vi "Main.vi"() -> ()   [LabVIEW 2024]
doc: "Aplikacja służąca do autoryzacji dostępu oparta na biometrycznej weryfikacji tożsamości"
uses:
  <vilib>/userDefined/High Color/IMAQdx.ctl
  <vilib>/vision/Image Controls.llb/IMAQ Image.ctl
  <vilib>/vision/driver/NI_Vision_Acquisition_Software.lvlib
panel:
  in  "Exit Application":bool caption="Click to terminate the application"
  in  "Tab Control":enum32{"Page 1", "Page 2", "Page 3", "Page 4"}(tab)
  in  "OK Button":bool
  out "Image Display":T1(plugin-control)
  in  "Input":string
  in  "Manage input data":bool
  in  "Add user":bool
  out "UserName":string
  out "Image Display 2":T1(plugin-control)
  in  "Save biometrics":bool
  in  "Name":string
  in  "Surname":string
  # "Processing..."
  # "Welcome"
  # "to control Panel"
  # "Now you can choose what you want to do"
  # "Simple input manager"
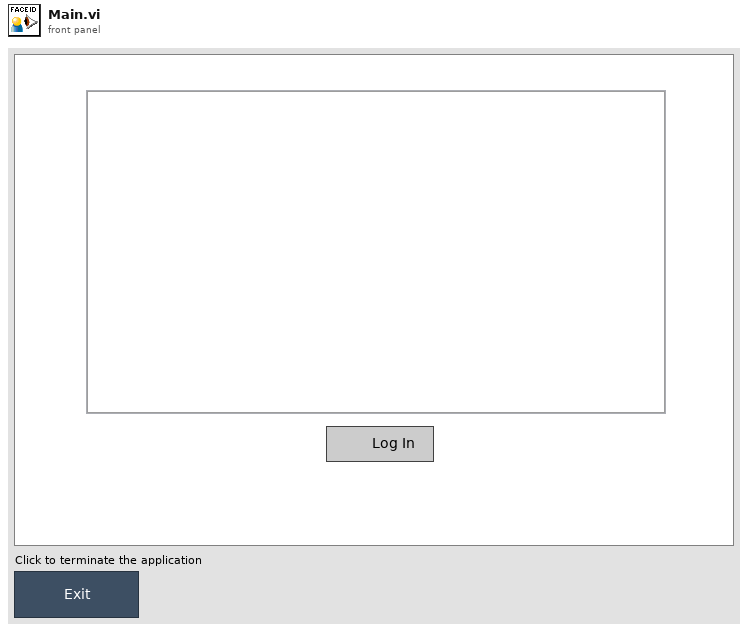
[diagram p1: front panel]
types:
  T1 = typedef "IMAQ Image.ctl" = refnum<image>
  T2 = enum32{"Invalid", "Standard", "Closed", "Hidden", "Minimized", "Maximized"}
  T3 = enum32{"invalid app kind", "Development System", "Run Time System", "Student Edition", "Embedded LabVIEW", "Evaluation", "Custom"}
  T4 = typedef "IMAQdx.ctl" = refnum<k21>
  T5 = cluster{"Core":cluster{"Current VI Reference":refnum<vi>, "Close Panel on Exit?":bool}, "New Image":T1, "IMAQdx Session":T4, "Img Path":string, "NameDisplay":string}
  T6 = cluster{"Current VI Reference":refnum<vi>, "Close Panel on Exit?":bool}
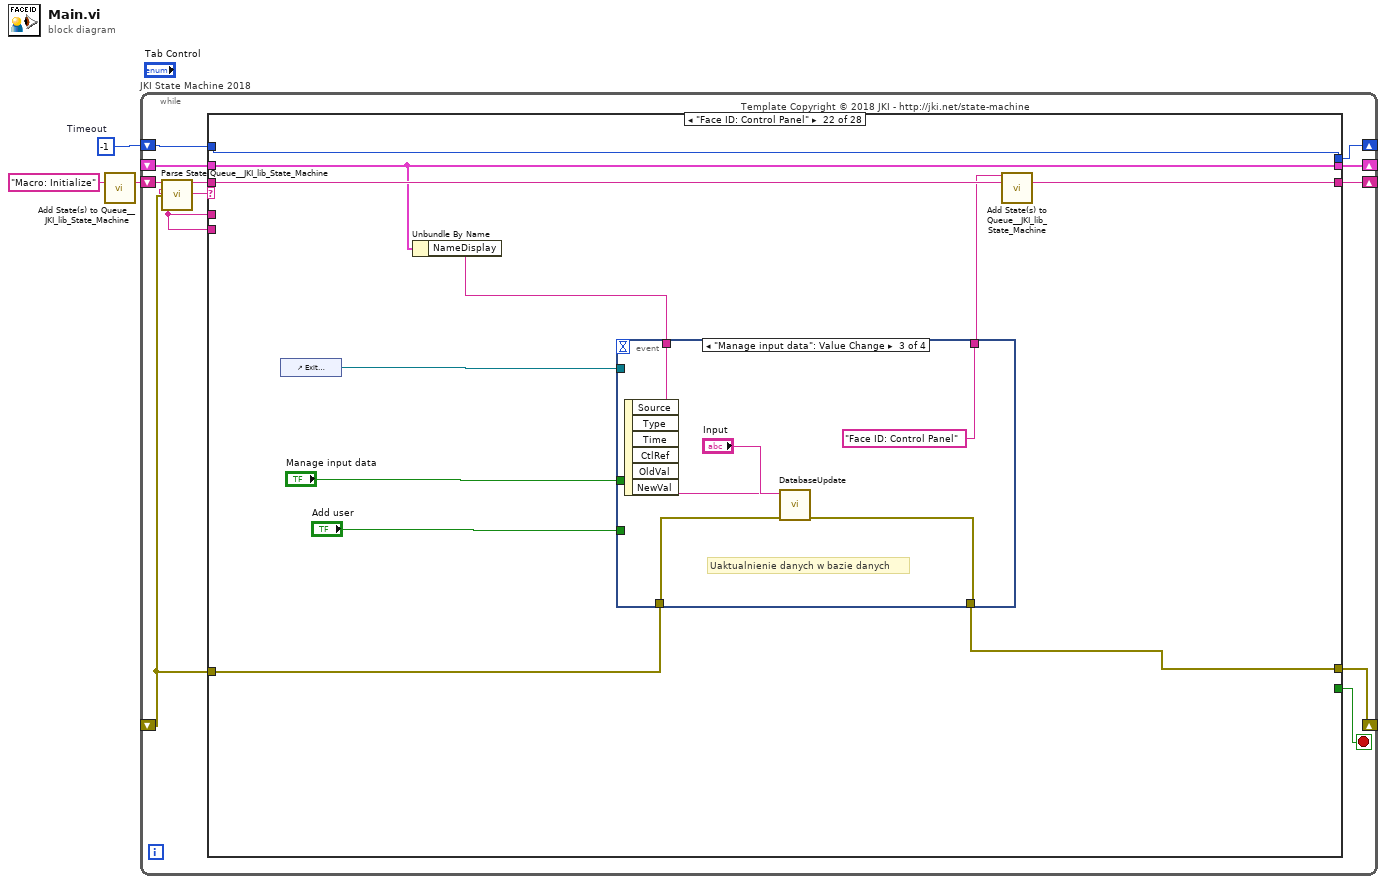
[diagram p0: block diagram]
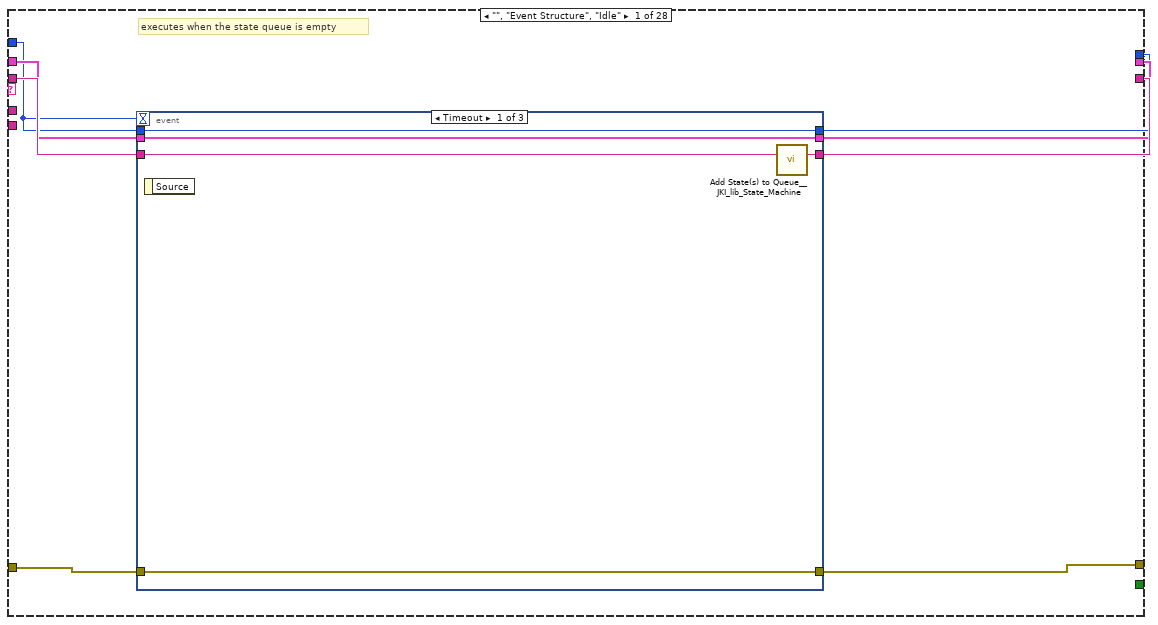
[diagram p2: hidden frame]
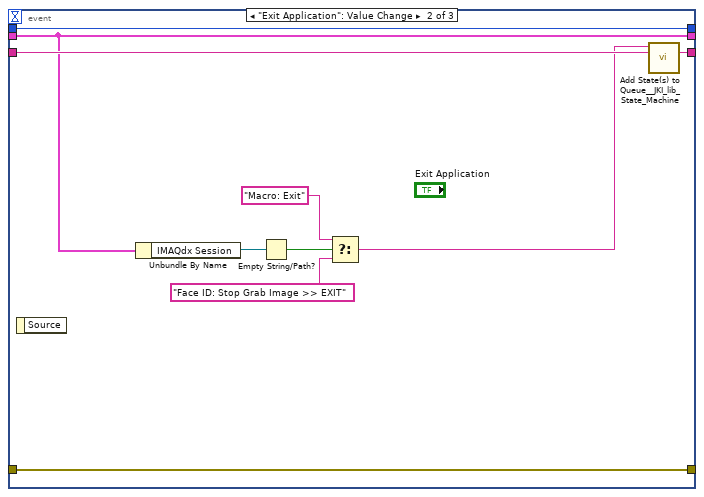
[diagram p3: hidden frame]
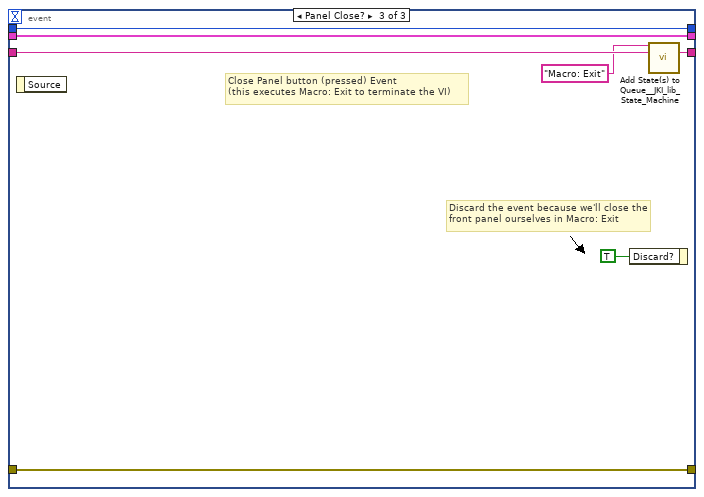
[diagram p4: hidden frame]
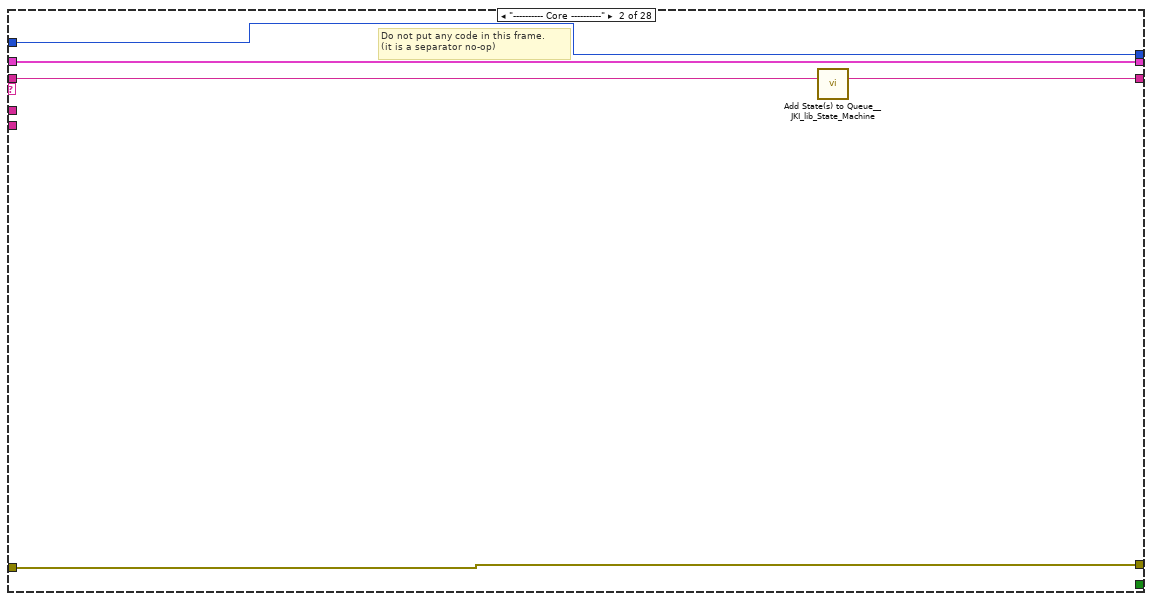
[diagram p5: hidden frame]
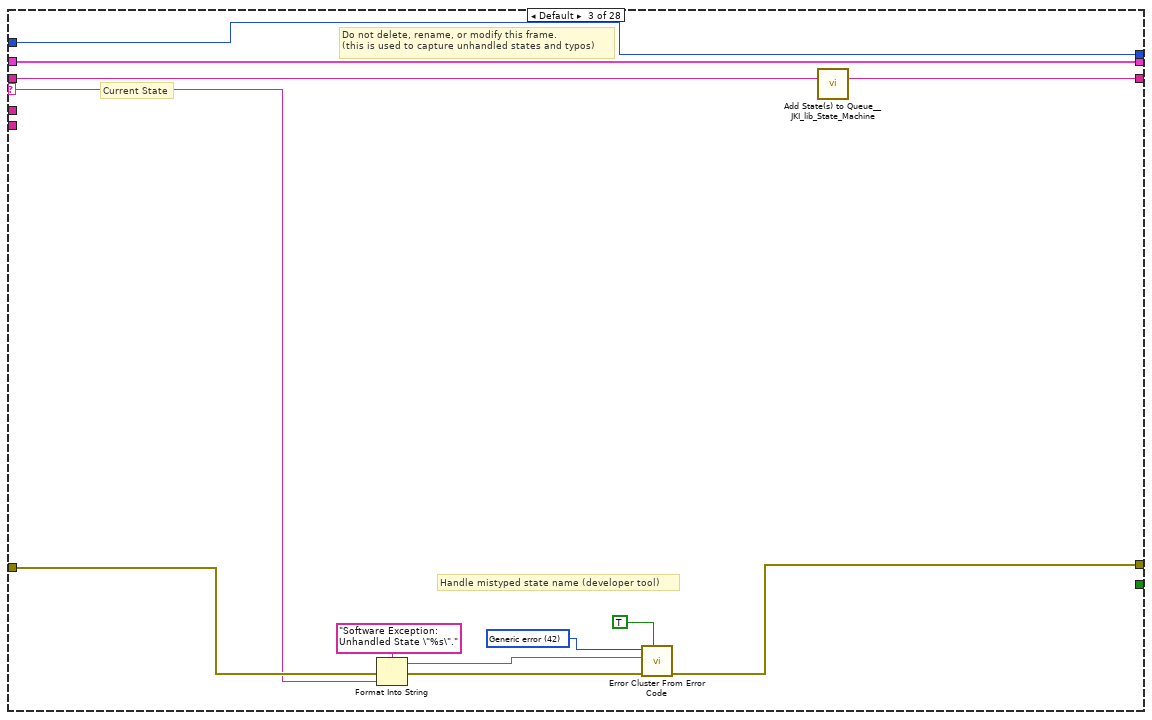
[diagram p6: hidden frame]
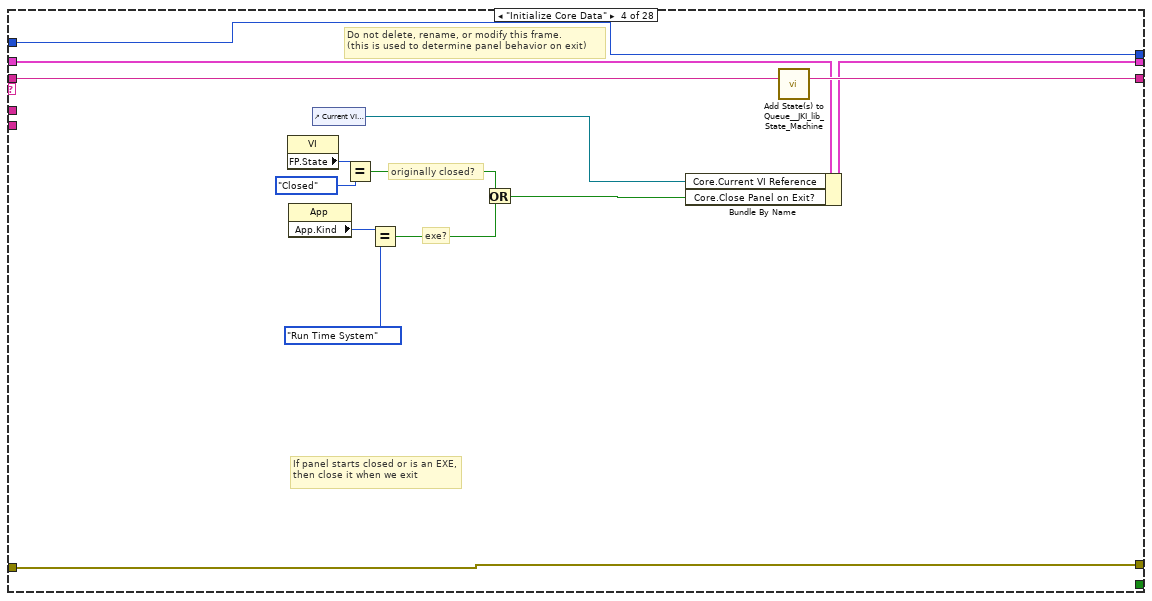
[diagram p7: hidden frame]
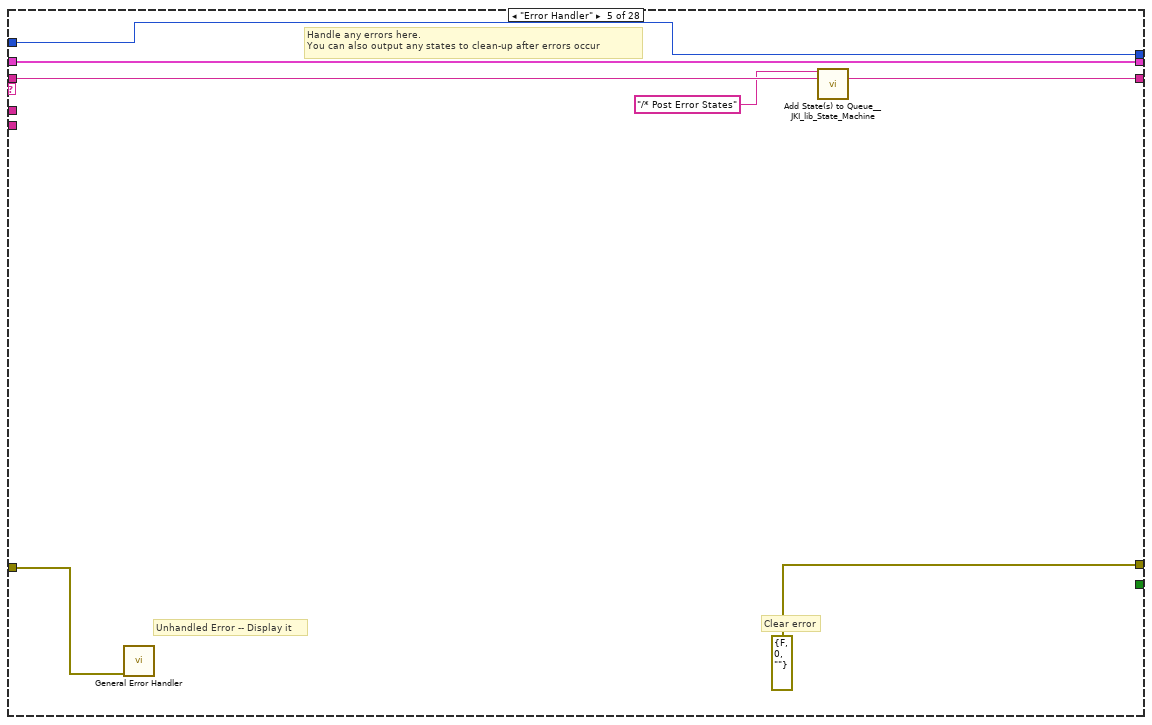
[diagram p8: hidden frame]
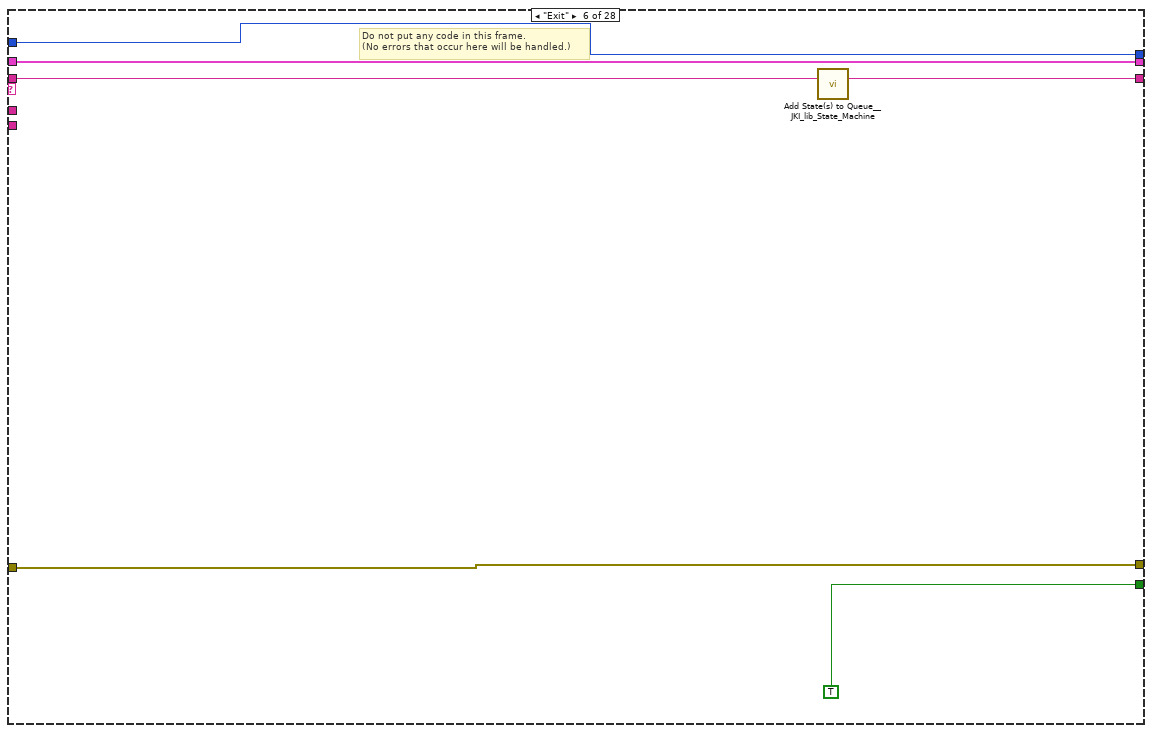
[diagram p9: hidden frame]
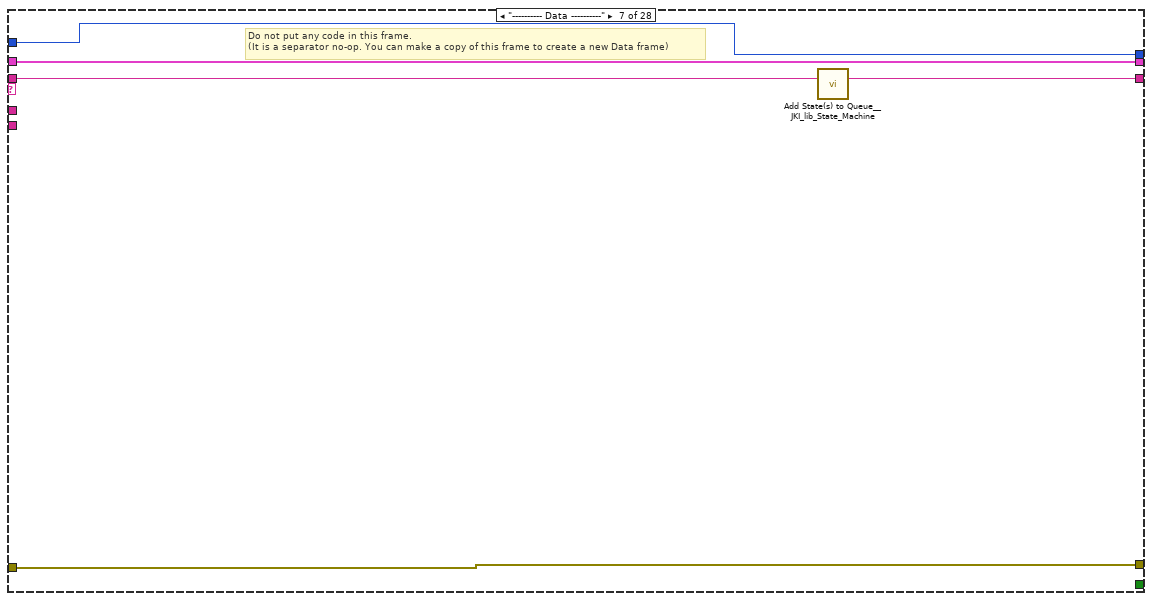
[diagram p10: hidden frame]
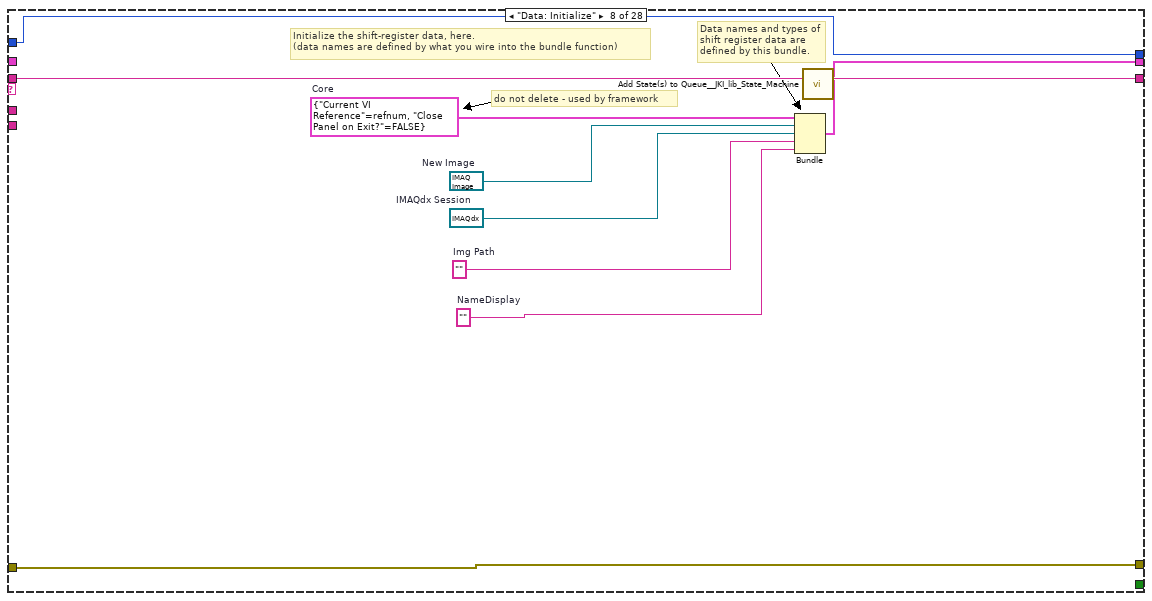
[diagram p11: hidden frame]
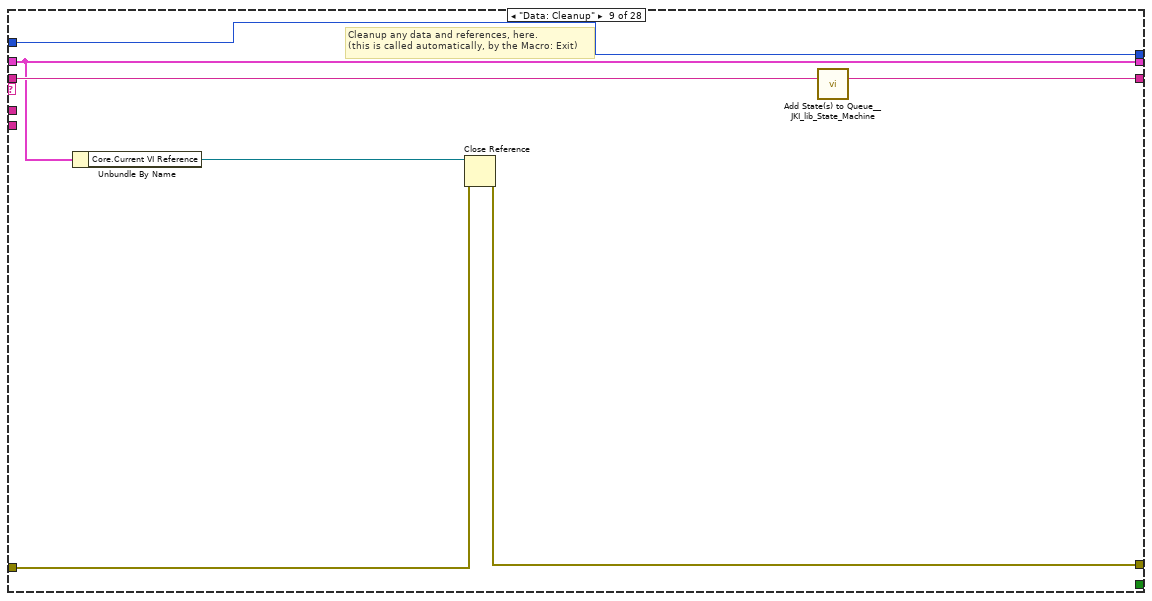
[diagram p12: hidden frame]
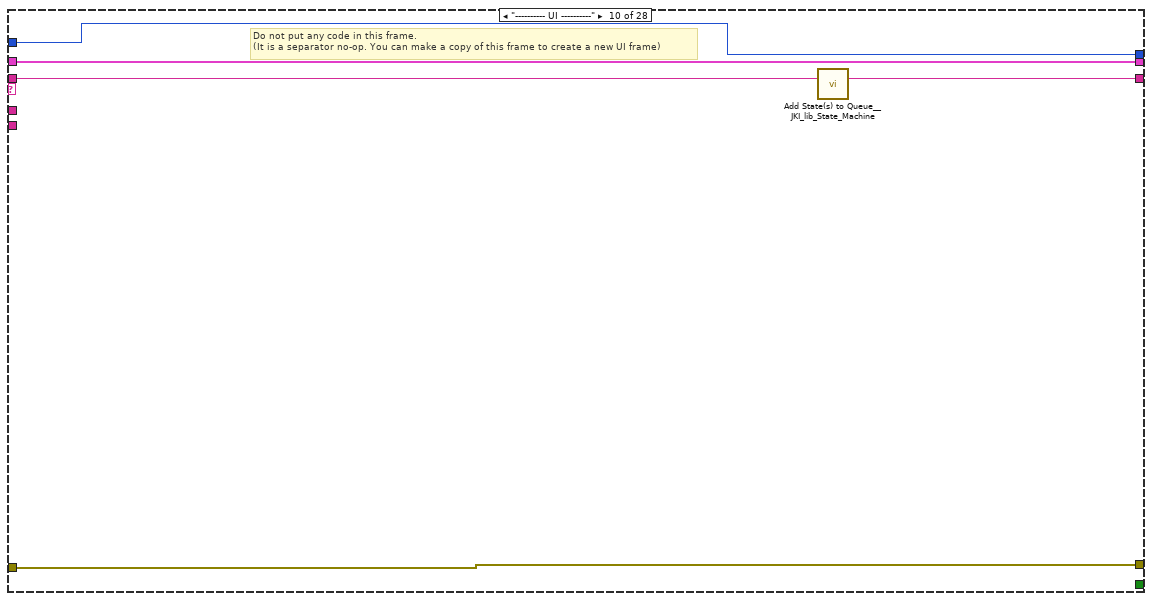
[diagram p13: hidden frame]
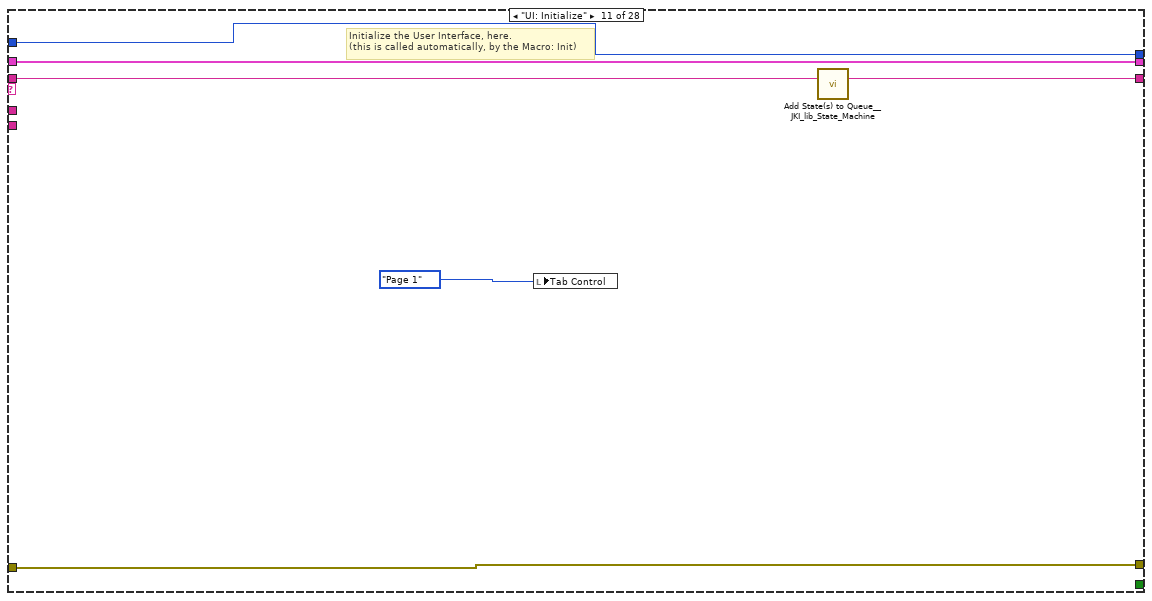
[diagram p14: hidden frame]
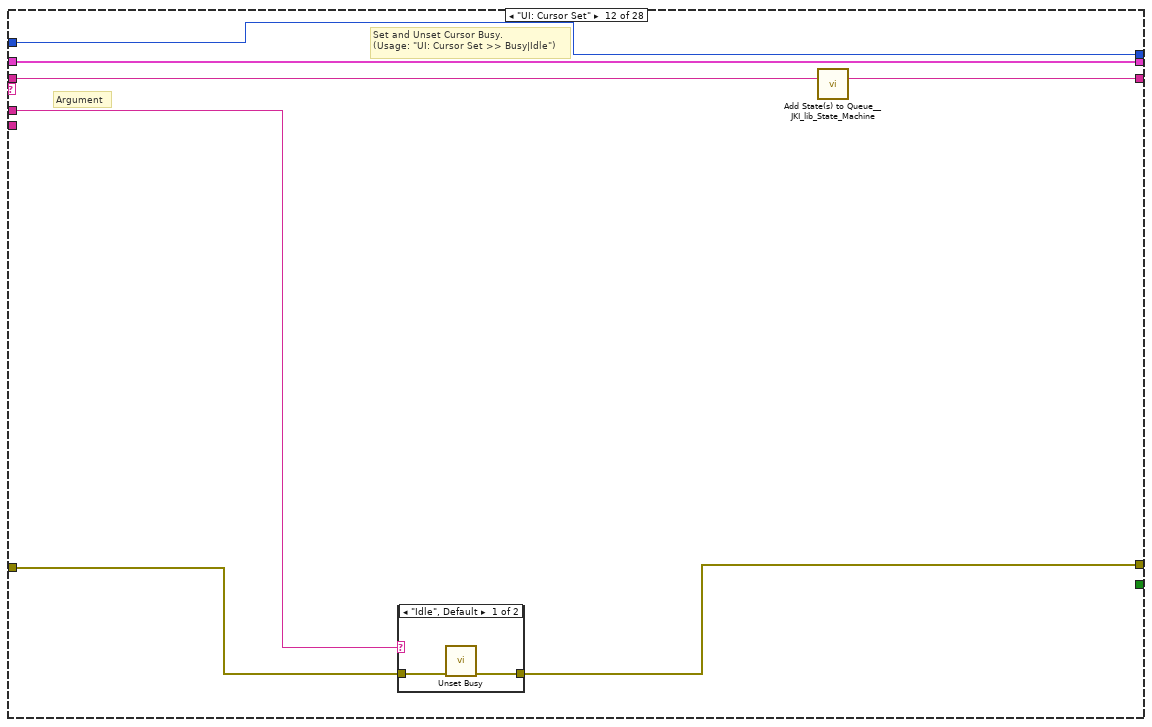
[diagram p15: hidden frame]
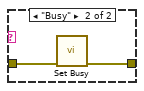
[diagram p16: hidden frame]
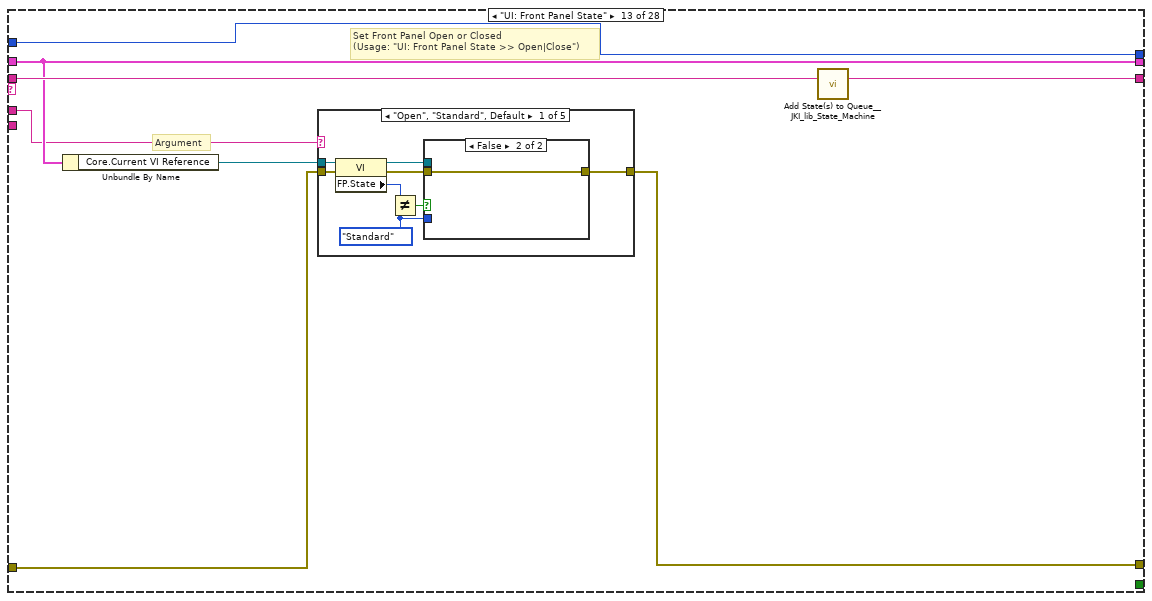
[diagram p17: hidden frame]
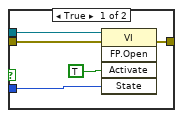
[diagram p18: hidden frame]
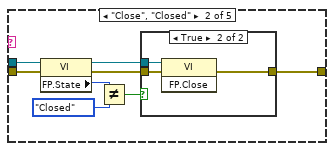
[diagram p19: hidden frame]
diagram:
  w1 = -1  # Timeout
  n1 = call <vilib>:"Add State(s) to Queue__JKI_lib_State_Machine.vi"("State(s) in (\"\")"="Macro: Initialize") -> ("States Out"=w3:string)  [unwired: 14 in]
  n2 = while "JKI State Machine 2018" {
    shift-right: [w9] -> _
    shift-left: _ -> [w8]
    shift-right: [w12] -> _
    shift-left: _ -> [w7]
    shift-right: [w11] -> _
    shift-left: w3 -> [w13]
    shift-right: [w5] -> _
    shift-left: w1 -> [w6]
    stop <- w10 stop-if-true
    # "Template Copyright © 2018 JKI - http://jki.net/state-machine"
    n3 = call <vilib>:"Parse State Queue__JKI_lib_State_Machine.vi"("State Queue"=w13, "Error In (no error)"=w7) -> ("Remaining States"=w14:string, "Current State"=w15:string, "Arguments"=w4:string)  [unwired: 11 in]
    n4 = case shown="\"Face ID: Control Panel\"" w15 {
      selector: w15 -> [_ _ w52 _ _ _ _ _ _ _ _ _ _ _ _ _ _ _ _ _ _ _ _ _ _ _ _ _]
      tunnel: w14 -> [w23 w50 w56 w76 w83 w89 w94 w104 w111 w116 w122 w129 w141 w211 w217 w228 w233 w241 w281 w306 w322 w338 w350 w355 w358 w367 w410 w428]
      tunnel: w4 -> [_ _ _ _ _ _ _ _ _ _ _ w124 w135 _ _ _ _ _ _ w287 _ _ _ _ _ _ _ _]
      tunnel: w8 -> [w21 w47 w54 w69 w80 w84 w91 _ w106 w113 w120 w127 w137 w208 w214 w225 w230 w234 w278 w295 w307 w334 w351 w354 w359 w362 w411 w429]
      tunnel: [w16 w48 w58 w73 errorcluster {"status"=FALSE, "code"=0, "source"=""} ("error out") w87 w92 w101 w107 w114 w119 w125 w138 w209 w215 w226 w231 w243 w273 w292 w311 w330 w349 w353 w357 w365 w401 w427] -> w12
      tunnel: w7 -> [w20 w48 w57 w73 w79 w87 w92 w101 w108 w114 w119 w126 w139 w209 w215 w226 w231 w242 w274 w299 w319 w332 w349 w353 w357 w366 w409 w419]
      tunnel: [w22 w49 w55 w75 w82 w88 w93 w103 w110 w115 w121 w128 w140 w210 w216 w227 w232 w251 w280 w305 w321 w339 w350 w355 w358 w364 w413 w424] -> w11
      tunnel: [_ _ _ _ _ TRUE _ _ _ _ _ _ _ _ _ _ _ _ _ _ _ _ _ _ _ _ _ _] -> w10
      tunnel: [w19 w47 w54 w74 w80 w84 w91 w102 w106 w113 w120 w127 w137 w208 w214 w225 w230 w235 w279 w296 w308 w334 w351 w354 w359 w361 w412 w425] -> w9
      tunnel: w6 -> [w18 w46 w51 w63 w77 w85 w90 w97 w105 w112 w118 w123 w134 w207 w212 w219 w229 w236 w277 _ w323 w340 w352 w356 w360 w368 w418 _]
      tunnel: [w17 w46 w51 w63 w77 w85 w90 w97 w105 w112 w118 w123 w134 w207 w212 w219 w229 w237 w277 -1 ("Timeout") w323 w340 w352 w356 w360 w363 w418 -1 ("Timeout")] -> w5
      tunnel: w4 -> [_ _ _ _ _ _ _ _ _ _ _ _ _ _ _ _ _ _ _ _ _ _ _ _ _ _ _ _]
      frame "", "Event Structure", "Idle" {
        # "executes when the state queue is empty"
        n5 = event shown="[0] Timeout" {
          selector: _ -> [_ _ _]
          dyn-events: _ -> [_ _ _]
          timeout: w18 -> [_ _ _]
          tunnel: w23 -> [w28 w38 w45]
          tunnel: [w27 w37 w44] -> w22
          tunnel: w21 -> [w25 w33 w42]
          tunnel: [w26 w36 w43] -> w16
          tunnel: w20 -> [w26 w36 w43]
          tunnel: [w25 w33 w42] -> w19
          tunnel: w18 -> [w24 w35 w39]
          tunnel: [w24 w35 w39] -> w17
          event Timeout {
            n6 = event-data() -> ()  [unwired: 1 in, 1 out]
            n7 = call <vilib>:"Add State(s) to Queue__JKI_lib_State_Machine.vi"("State(s) in (\"\")"=w28) -> ("States Out"=w27:string)  [unwired: 14 in]
          }
          event "Exit Application": Value Change {
            n8 = event-data() -> ()  [unwired: 1 in, 1 out]
            n9 = Unbundle By Name(w33) -> ("IMAQdx Session"=w34:T4)
            n10 = Empty String/Path?(string/path=w34) -> (empty?=w32:bool)
            n11 = Select(t="Macro: Exit", s=w32, f="Face ID: Stop Grab Image >> EXIT") -> (s? t:f=w31:string)
            n12 = call <vilib>:"Add State(s) to Queue__JKI_lib_State_Machine.vi"("State(s) in Front (\"\")"=w31, "State(s) in (\"\")"=w38) -> ("States Out"=w37:string)  [unwired: 13 in]
          }
          event Panel Close? {
            # "Discard the event because we'll close the front panel ourselves in Macro: Exit"
            # "Close Panel button (pressed) Event\n(this executes Macro: Exit to terminate the VI)"
            n13 = event-data() -> ()  [unwired: 1 in, 1 out]
            n14 = event-data("Discard?"=TRUE) -> ()  [unwired: 1 in, 1 out]
            n15 = call <vilib>:"Add State(s) to Queue__JKI_lib_State_Machine.vi"("State(s) in Front (\"\")"="Macro: Exit", "State(s) in (\"\")"=w45) -> ("States Out"=w44:string)  [unwired: 13 in]
          }
        }
      }
      frame "---------- Core ----------" {
        # "Do not put any code in this frame.\n(it is a separator no-op)"
        n16 = call <vilib>:"Add State(s) to Queue__JKI_lib_State_Machine.vi"("State(s) in (\"\")"=w50) -> ("States Out"=w49:string)  [unwired: 14 in]
      }
      frame Default {
        w61 = 42 items=["No error", "Argument error", "Memory is full", "Out of zone", "End of file", "File already open", "Generic file I/O error", "File not found", "File permission error", "Disk is full", "Duplicate path", "Too many files open", "System feature not enabled", "Resource file not found", "Cannot add resource", "Resource not found", "Image not found", "Image memory error", "Pen does not exist", "Config type invalid", "Config token not found", "Config parse error", "Config memory error", "Bad external code format", "Bad external code offset", "External code not present", "Null window", "Destroy window error", "Null menu", "Print aborted", "Bad print record", "Print driver error", "Windows error during printing", "Memory error during printing", "Print dialog error", "Generic print error", "Invalid device refnum", "Device not found", "Device parameter error", "Device unit error", "Cannot open device", "Device call aborted", "Generic error", "Cancelled by user", "Object ID too low", "Object ID too high", "Object not in heap", "Unknown heap", "Unknown object (invalid DefProc)", "Unknown object (DefProc not in table)", "Message out of range", "Invalid (null) method", "Unknown message", "Manager call not supported", "Bad address", "Network operation in progress", "Network operation timed out", "Connection is busy", "Network attribute not supported", "Network error", "Address in use", "System out of memory", "Connection aborted", "Connection refused", "Not connected", "Already connected", "Connection closed", "Initialization error (interapplication manager)", "Bad occurrence", "Wait on unbound occurrence handler", "Occurrence queue overflow", "Datalog type conflict", "Unused", "Unrecognized type (interapplication manager)", "Memory corrupt", "Failed to make temporary DLL", "Old CIN version", "Drag socket not found", "Failed to load drop-object", "Failed to register OLE object", "Failed to release OLE object", "Format specifier type mismatch", "Unknown format specifier", "Too few format specifiers", "Too many format specifiers", "Scan failed", "Newer CIN version", "Error converting to variant", "Runtime menu error", "Password tampered", "Variant attribute not found", "Incompatible variant data type", "Event data is not available", "Event Store is not present", "Occurrence is not found", "Event Queue is not created", "Event info is not available", "Refnum passed is NULL", "Error retrieving Class GUID", "Error retrieving CoClass GUID", "Error retrieving TypeLib GUID.", "Bad built application magic bytes.", "Specific driver is different from the specific driver associated with the Logical Name.", "There is no session opened to the class driver.", "Max Error", "MAX - Error with config objects", "MAX - Error loading configuration", "MAX - Group not supported"]
        # "Current State"
        # "Do not delete, rename, or modify this frame.\n(this is used to capture unhandled states and typos)"
        # "Handle mistyped state name (developer tool)"
        n17 = Format Into String(format string="Software Exception: Unhandled State \"%s\"." ("message"), error in=w57, w52) -> (resulting string=w60:string, error out=w59:errorcluster)  [unwired: 1 in]
        n18 = call <vilib>:"Error Cluster From Error Code.vi"("show call chain? (False)"=TRUE, "error in (no error)"=w59, "error message (\"\")"=w60, "error code (0)"=w61) -> ("error out"=w58:errorcluster)  [unwired: 5 in]
        n19 = call <vilib>:"Add State(s) to Queue__JKI_lib_State_Machine.vi"("State(s) in (\"\")"=w56) -> ("States Out"=w55:string)  [unwired: 14 in]
      }
      frame "Initialize Core Data" {
        # "Do not delete, rename, or modify this frame.\n(this is used to determine panel behavior on exit)"
        # "originally closed?"
        # "exe?"
        # "If panel starts closed or is an EXE, then close it when we exit"
        n20 = property class="VI"() -> ("FP.State"=w66:T2)  [unwired: 2 in, 2 out]
        n21 = property class="App"() -> ("App.Kind"=w72:T3)  [unwired: 2 in, 2 out]
        n22 = control-ref of="Current VI Reference"() -> (w67:refnum<vi>)
        n23 = Equal?(x=w66, y=T2."Closed" ("Front Panel Window:State")) -> (x = y?=w64:bool)
        n24 = Equal?(x=w72, y=T3."Run Time System" ("Application:Kind")) -> (x = y?=w70:bool)
        n25 = Or(x=w64, y=w70) -> (x .or. y?=w68:bool)
        n26 = Bundle By Name(cluster=w69, "Core.Current VI Reference"=w67, "Core.Close Panel on Exit?"=w68) -> (w74:T5)
        n27 = call <vilib>:"Add State(s) to Queue__JKI_lib_State_Machine.vi"("State(s) in (\"\")"=w76) -> ("States Out"=w75:string)  [unwired: 14 in]
      }
      frame "Error Handler" {
        # "Unhandled Error -- Display it"
        # "Handle any errors here.\nYou can also output any states to clean-up after errors occur"
        # "Clear error"
        n28 = call <vilib>:"General Error Handler.vi"("error in (no error)"=w79) -> ()  [unwired: 10 in, 5 out]
        n29 = call <vilib>:"Add State(s) to Queue__JKI_lib_State_Machine.vi"("State(s) in Front (\"\")"="/* Post Error States", "State(s) in (\"\")"=w83) -> ("States Out"=w82:string)  [unwired: 13 in]
      }
      frame "Exit" {
        # "Do not put any code in this frame.\n(No errors that occur here will be handled.)"
        n30 = call <vilib>:"Add State(s) to Queue__JKI_lib_State_Machine.vi"("State(s) in (\"\")"=w89) -> ("States Out"=w88:string)  [unwired: 14 in]
      }
      frame "---------- Data ----------" {
        # "Do not put any code in this frame.\n(It is a separator no-op. You can make a copy of this frame to create a new Data frame)"
        n31 = call <vilib>:"Add State(s) to Queue__JKI_lib_State_Machine.vi"("State(s) in (\"\")"=w94) -> ("States Out"=w93:string)  [unwired: 14 in]
      }
      frame "Data: Initialize" {
        w95 = ""  # NameDisplay
        w96 = ""  # Img Path
        w98 = T1 refnum  # New Image
        w99 = T4 refnum  # IMAQdx Session
        w100 = T6 {"Current VI Reference"=refnum, "Close Panel on Exit?"=FALSE}  # Core
        # "do not delete - used by framework"
        # "Data names and types of shift register data are defined by this bundle."
        # "Initialize the shift-register data, here.\n(data names are defined by what you wire into the bundle function)"
        n32 = Bundle("Core"=w100, "New Image"=w98, "IMAQdx Session"=w99, "Img Path"=w96, "NameDisplay"=w95) -> (w102:T5)  [unwired: 1 in]
        n33 = call <vilib>:"Add State(s) to Queue__JKI_lib_State_Machine.vi"("State(s) in (\"\")"=w104) -> ("States Out"=w103:string)  [unwired: 14 in]
      }
      frame "Data: Cleanup" {
        # "Cleanup any data and references, here.\n(this is called automatically, by the Macro: Exit)"
        n34 = Unbundle By Name(w106) -> ("Core.Current VI Reference"=w109:refnum<vi>)
        n35 = Close Reference(reference=w109, error in (no error)=w108) -> (error out=w107:errorcluster)
        n36 = call <vilib>:"Add State(s) to Queue__JKI_lib_State_Machine.vi"("State(s) in (\"\")"=w111) -> ("States Out"=w110:string)  [unwired: 14 in]
      }
      frame "---------- UI ----------" {
        # "Do not put any code in this frame.\n(It is a separator no-op. You can make a copy of this frame to create a new UI frame)"
        n37 = call <vilib>:"Add State(s) to Queue__JKI_lib_State_Machine.vi"("State(s) in (\"\")"=w116) -> ("States Out"=w115:string)  [unwired: 14 in]
      }
      frame "UI: Initialize" {
        # "Initialize the User Interface, here.\n(this is called automatically, by the Macro: Init)"
        n38 = local write "Tab Control"(enum32{"Page 1", "Page 2", "Page 3", "Page 4"}."Page 1" ("Tab Control")) -> ()
        n39 = call <vilib>:"Add State(s) to Queue__JKI_lib_State_Machine.vi"("State(s) in (\"\")"=w122) -> ("States Out"=w121:string)  [unwired: 14 in]
      }
      frame "UI: Cursor Set" {
        # "Argument"
        # "Set and Unset Cursor Busy.\n(Usage: \"UI: Cursor Set >> Busy|Idle\")"
        n40 = case shown="\"Idle\", Default" w124 {
          tunnel: w126 -> [w131 w133]
          tunnel: [w130 w132] -> w125
          frame "Idle", Default {
            n41 = call <vilib>:"Unset Busy.vi"("error in (no error)"=w131) -> ("error out"=w130:errorcluster)  [unwired: 10 in]
          }
          frame "Busy" {
            n42 = call <vilib>:"Set Busy.vi"("error in (no error)"=w133) -> ("error out"=w132:errorcluster)  [unwired: 9 in, 1 out]
          }
        }
        n43 = call <vilib>:"Add State(s) to Queue__JKI_lib_State_Machine.vi"("State(s) in (\"\")"=w129) -> ("States Out"=w128:string)  [unwired: 14 in]
      }
      frame "UI: Front Panel State" {
        # "Argument"
        # "Set Front Panel Open or Closed\n(Usage: \"UI: Front Panel State >> Open|Close\")"
        n44 = Unbundle By Name(w137) -> ("Core.Current VI Reference"=w136:refnum<vi>)
        n45 = case shown="\"Open\", \"Standard\", Default" w135 {
          tunnel: w139 -> [w147 w162 w173 w186 w199]
          tunnel: [w149 w163 w175 w188 w201] -> w138
          tunnel: w136 -> [w148 w160 w174 w187 w200]
          frame "Open", "Standard", Default {
            w142 = T2."Standard" ("State")
            n46 = property class="VI"(reference=w148, error in=w147) -> (reference out=w145:refnum<vi>, error out=w146:errorcluster, "FP.State"=w144:T2)
            n47 = Not Equal?(x=w144, y=w142) -> (x != y?=w143:bool)
            n48 = case shown="False" w143 {
              tunnel: [w153 w155] -> w149
              tunnel: w146 -> [w152 w155]
              tunnel: w145 -> [w151 _]
              tunnel: w142 -> [w150 _]
              frame True {
                n49 = invoke class="VI" method="FP.Open"(reference=w151, error in=w152, "Activate"=TRUE, "State"=w150) -> (error out=w153:errorcluster)  [unwired: 1 in, 4 out]
              }
              frame False {
              }
            }
          }
          frame "Close", "Closed" {
            n50 = property class="VI"(reference=w160, error in=w162) -> (reference out=w159:refnum<vi>, error out=w161:errorcluster, "FP.State"=w157:T2)
            n51 = Not Equal?(x=w157, y=T2."Closed" ("Front Panel Window:State")) -> (x != y?=w156:bool)
            n52 = case shown="True" w156 {
              tunnel: [w164 w167] -> w163
              tunnel: w161 -> [w164 w166]
              tunnel: w159 -> [_ w165]
              frame False {
              }
              frame True {
                n53 = invoke class="VI" method="FP.Close"(reference=w165, error in=w166) -> (error out=w167:errorcluster)  [unwired: 1 in, 2 out]
              }
            }
          }
          frame "Hidden", "Hide" {
            w168 = T2."Hidden" ("State")
            n54 = property class="VI"(reference=w174, error in=w173) -> (reference out=w171:refnum<vi>, error out=w172:errorcluster, "FP.State"=w170:T2)
            n55 = Not Equal?(x=w170, y=w168) -> (x != y?=w169:bool)
            n56 = case shown="True" w169 {
              tunnel: [w179 w180] -> w175
              tunnel: w172 -> [w178 w180]
              tunnel: w171 -> [w177 _]
              tunnel: w168 -> [w176 _]
              frame True {
                n57 = invoke class="VI" method="FP.Open"(reference=w177, error in=w178, "State"=w176) -> (error out=w179:errorcluster)  [unwired: 2 in, 4 out]
              }
              frame False {
              }
            }
          }
          frame "Minimize", "Minimized" {
            w181 = T2."Minimized" ("State")
            n58 = property class="VI"(reference=w187, error in=w186) -> (reference out=w184:refnum<vi>, error out=w185:errorcluster, "FP.State"=w183:T2)
            n59 = Not Equal?(x=w183, y=w181) -> (x != y?=w182:bool)
            n60 = case shown="True" w182 {
              tunnel: [w192 w193] -> w188
              tunnel: w185 -> [w191 w193]
              tunnel: w184 -> [w190 _]
              tunnel: w181 -> [w189 _]
              frame True {
                n61 = invoke class="VI" method="FP.Open"(reference=w190, error in=w191, "State"=w189) -> (error out=w192:errorcluster)  [unwired: 2 in, 4 out]
              }
              frame False {
              }
            }
          }
          frame "Maximize", "Maximized" {
            w194 = T2."Maximized" ("State")
            n62 = property class="VI"(reference=w200, error in=w199) -> (reference out=w197:refnum<vi>, error out=w198:errorcluster, "FP.State"=w196:T2)
            n63 = Not Equal?(x=w196, y=w194) -> (x != y?=w195:bool)
            n64 = case shown="True" w195 {
              tunnel: [w205 w206] -> w201
              tunnel: w198 -> [w204 w206]
              tunnel: w197 -> [w203 _]
              tunnel: w194 -> [w202 _]
              frame True {
                n65 = invoke class="VI" method="FP.Open"(reference=w203, error in=w204, "State"=w202) -> (error out=w205:errorcluster)  [unwired: 2 in, 4 out]
              }
              frame False {
              }
            }
          }
        }
        n66 = call <vilib>:"Add State(s) to Queue__JKI_lib_State_Machine.vi"("State(s) in (\"\")"=w141) -> ("States Out"=w140:string)  [unwired: 14 in]
      }
      frame "---------- Macro ----------" {
        # "Do not put any code in this frame.\n(It is a separator no-op. You can make a copy of this frame to create a new Macro frame)"
        n67 = call <vilib>:"Add State(s) to Queue__JKI_lib_State_Machine.vi"("State(s) in (\"\")"=w211) -> ("States Out"=w210:string)  [unwired: 14 in]
      }
      frame "Macro: Initialize" {
        w213 = "Data: Initialize\nInitialize Core Data\nUI: Initialize\nUI: Front Panel State >> Open\nFace ID: Initialize Grab Image"  # Data: Initialize Initialize Core Data UI: Initialize UI: Front Panel State >> Open Face ID: Initialize Grab Image
        # "Initialization Macro\n(This is called once, when the VI starts)"
        n68 = call <vilib>:"Add State(s) to Queue__JKI_lib_State_Machine.vi"("State(s) in Front (\"\")"=w213, "State(s) in (\"\")"=w217) -> ("States Out"=w216:string)  [unwired: 13 in]
      }
      frame "Macro: Exit" {
        # "Exit Macro\n(This is called once, when the VI exits)"
        n69 = Unbundle By Name(w225) -> ("Core.Close Panel on Exit?"=w224:bool)
        n70 = Select(t="UI: Front Panel State >> Close", s=w224, f="") -> (s? t:f=w221:string)
        n71 = call <vilib>:"Add State(s) to Queue__JKI_lib_State_Machine.vi"("State(s) in (\"\")"=w221, "State(s) at Back (\"\")"="Data: Cleanup\nExit") -> ("States Out"=w220:string)  [unwired: 13 in]
        n72 = call <vilib>:"Add State(s) to Queue__JKI_lib_State_Machine.vi"("State(s) in Front (\"\")"=w220, "State(s) in (\"\")"=w228) -> ("States Out"=w227:string)  [unwired: 13 in]
      }
      frame "---------- Face ID ----------" {
        # "Template Separator\n(You can make a copy of, or modify, this frame)"
        n73 = call <vilib>:"Add State(s) to Queue__JKI_lib_State_Machine.vi"("State(s) in (\"\")"=w233) -> ("States Out"=w232:string)  [unwired: 14 in]
      }
      frame "Face ID: Initialize Grab Image" {
        # "Korzystając z bloku \"Bundle by Name\" tworzony jest klaster złożony z referencji do obrazu oraz sesji kamery.\nDane te są przesyłane do kolejnych stanów za pomocą linii \"Data Wire\""
        # "Po zatwierdzeniu wyboru kamery blok sprawdza poprawność i dostępność kamery - na tej podstawie wykonuje się odpowiedni Case struktury"
        # "/// Blok opcjonalny\nWyświetla i pozwala wybrać jedną z dostępnych kamer"
        n74 = call "List Available Cameras.vi"("error in"=w242) -> ("error out"=w248:errorcluster, "VendorName"=w249:string[], "Available Cameras"=w250:string[])  [unwired: 8 in]
        n75 = call "Select Camera Dialog.vi"("error in (no error)"=w248, "Vendor Name"=w249, "Camera Name"=w250) -> ("error out"=w244:errorcluster, "No camera?"=w247:bool, "Interface Name"=w246:string)  [unwired: 6 in]
        n76 = case shown="True" w247 {
          tunnel: w246 -> [w262 _]
          tunnel: [w260 T4 refnum ("Session Out")] -> w245
          tunnel: w244 -> [w258 w267]
          tunnel: [w257 w267] -> w243
          tunnel: w241 -> [w256 _]
          tunnel: [w256 w265] -> w240
          tunnel: [w254 T1 refnum ("New Image")] -> w239
          tunnel: ["Face ID: Grab Image" ("Remaining States") w265] -> w238
          tunnel: [10 w264] -> w237
          tunnel: w236 -> [_ w264]
          frame False {
            w263 = u32 5  # Number of Buffers
            # "Blok biblioteki IMAQdx \"Configure Grab\" konfiguruje akwizycję obrazów"
            # "Blok biblioteki IMAQdx \"Open Camera\" konfiguruje kamerę"
            # "Jeśli kamera została poprawnie zainicjalizowana na kolejne zostaje dodany stan: \"Face ID: Grab Image\""
            # "Aby uniknąć zawieszenia aplikacji w stanie \"Event Structure\", \"Idle\" generujemy Timeout"
            # "Tworzenie referencji do przechowywania obrazu w pamięci komputera"
            n77 = call <vilib>:"IMAQdx Open Camera.vi"("error in"=w258, "Session In"=w262) -> ("error out"=w259:errorcluster, "Session Out"=w261:T4)  [unwired: 1 in, 7 out]
            n78 = call <vilib>:"IMAQdx Configure Grab.vi"("error in"=w259, "Number of Buffers"=w263, "Session In"=w261) -> ("error out"=w257:errorcluster, "Session Out"=w260:T4)  [unwired: 7 in]
            n79 = call "IMAQ Create"("Image Name"="Acquire Most Recent Image") -> ("New Image"=w254:T1)  [unwired: 3 in, 2 out]
          }
          frame True {
            w265 = ""
            # "Pusta sesja kamery"
            # "Pusta referencja do obrazu"
            # "W razie wystąpienia błędu inicjalizacji kamery zostanie wygenerowany błąd z kodem: -1074360311"
            # "Usuwane są wszystkie kolejne stany z kolejki.\nProgram przechodzi do stanu \"Error Handler\""
            # "Camera not found"
          }
        }
        n80 = Bundle By Name(cluster=w234, "New Image"=w239, "IMAQdx Session"=w245) -> (w235:T5)
        n81 = call <vilib>:"Add State(s) to Queue__JKI_lib_State_Machine.vi"("State(s) in Front (\"\")"=w238, "State(s) in (\"\")"=w240) -> ("States Out"=w251:string)  [unwired: 13 in]
      }
      frame "Face ID: Grab Image" {
        # "Przycisk odpowiedzialny za rozpoczęcie procesu logowania"
        # "Korzystając z bloku \"Bundle by Name\" tworzony jest klaster złożony z referencji do obrazu oraz sesji kamery.\nDane te są przesyłane do kolejnych stanów za pomocą linii \"Data Wire\""
        # "Blok odpowiadający za wyświetlenie pobranego obrazu na ekranie"
        # "SubVi \"Take Image Case Struct\" odpowiada za właściwą akwizycję obrazu. \nDodatkowe komentarze znajdują się w SubVi."
        # "Z linii \"Data Wire\" pobierane zostają ( \"rozpakowane\" za pomocną bloku \"Unbundle by Name\" referencja do obrazu oraz aktualna sesja kamery"
        n82 = Unbundle By Name(w278) -> ("IMAQdx Session"=w276:T4, "New Image"=w275:T1)
        n83 = call "Take Image Case Struct.vi"("error in (no error)"=w274, "OK Button"="OK Button", "Image In"=w275, "Session In"=w276) -> ("error out"=w273:errorcluster, "State"=w271:string, "Image Out"=w270:T1, "Session Out"=w272:T4)  [unwired: 4 in]
        "Image Display" <- w270
        n84 = Bundle By Name(cluster=w278, "IMAQdx Session"=w272, "New Image"=w270) -> (w279:T5)
        n85 = call <vilib>:"Add State(s) to Queue__JKI_lib_State_Machine.vi"("State(s) in Front (\"\")"=w271, "State(s) in (\"\")"=w281) -> ("States Out"=w280:string)  [unwired: 13 in]
      }
      frame "Face ID: Stop Grab Image" {
        # "Usunięcie referencji z pamięci komputera do obrazu pobranego podczas procesu logowania."
        # "Blok odpowiedzialny za zapis obrazu do pliku w formacie JPEG. \nFormat pliku można wybrać z rozwijnej listy typu wyliczeniowego."
        # "Sekwencja bloków odpowiedzialna za zatrzymanie akwizycji obrazu oraz usunięcia referencji do kamery z pamięci komputera"
        # "Pobieranie ścieżki do aktualnego folderu w którym znajduje się Vi"
        # "Tworzenie ścieżki do pliku za pomocą ścieżeki względnej w połączeniu z ścieżką do pliku tymczasowego"
        # "Dodanie do kolejki stanu \"Face ID: Image Processing\" w celu analizy pobranego obrazu"
        # "Korzystając z bloku \"Bundle by Name\" tworzony jest klaster złożony z sesji kamery.\nDane te są przesyłane do kolejnych stanów za pomocą linii \"Data Wire\""
        # "Wyłączenie timeout-u"
        # "Sukces! Wykryli[my twarz, lecimy dalej!"
        n86 = Unbundle By Name(w295) -> ("New Image"=w291:T1, "IMAQdx Session"=w300:T4)
        n87 = Current VI's Path() -> (path=w290:path)
        n88 = call <vilib>:"IMAQdx Stop Acquisition.vi"("error in"=w299, "Session In"=w300) -> ("error out"=w304:errorcluster, "Session Out"=w303:T4)  [unwired: 8 out]
        n89 = call <vilib>:"IMAQdx Unconfigure Acquisition.vi"("error in"=w304, "Session In"=w303) -> ("error out"=w301:errorcluster, "Session Out"=w302:T4)  [unwired: 8 out]
        n90 = Build Path(base path=w290, name or relative path=path "../Data/Log_temp_storage/log.jpg") -> (appended path=w288:path)
        n91 = call <vilib>:"IMAQdx Close Camera.vi"("error in"=w301, "Session In"=w302) -> ("error out"=w294:errorcluster)  [unwired: 9 out]
        n92 = call-poly "IMAQ Write File 2"("error in (no error)"=w294, "File Path"=w288, "Image"=w291) -> ("error out"=w293:errorcluster)  [unwired: 7 in, 1 out]
        n93 = Equal?(x=w287, y="EXIT") -> (x = y?=w285:bool)
        n94 = call "Imaq Dispose"("Image"=w291, "error in (no error)"=w293) -> ("error out"=w292:errorcluster)  [unwired: 4 in]
        n95 = Bundle By Name(cluster=w295, "IMAQdx Session"=T4 refnum) -> (w296:T5)
        n96 = Select(t="Macro: Exit", s=w285, f="Face ID: Image Processing") -> (s? t:f=w282:string)
        n97 = call <vilib>:"Add State(s) to Queue__JKI_lib_State_Machine.vi"("State(s) in Front (\"\")"=w282, "State(s) in (\"\")"=w306) -> ("States Out"=w305:string)  [unwired: 13 in]
      }
      frame "Face ID: Image Processing" {
        # "Przejście do kolejnej zakładki - ekranu przejściowego trwającego podczas analizy obrazu"
        n98 = Current VI's Path() -> (path=w318:path)
        n99 = Build Path(base path=w318, name or relative path=path "../Python Code/compare_faces_py.py") -> (appended path=w316:path)
        n100 = local write "Tab Control"(enum32{"Page 1", "Page 2", "Page 3", "Page 4"}."Page 2" ("Tab Control")) -> ()
        n101 = call "Python.vi"("error in (no error)"=w319, "module path"=w316) -> ("error out"=w312:errorcluster, "return value"=w310:string)  [unwired: 8 in]
        n102 = call "DatabaseRead SubVI.vi"("error in (no error)"=w312, "File name"=w310) -> ("error out"=w311:errorcluster, "UserName"=w309:string)  [unwired: 8 in]
        "UserName" <- w309
        n103 = Not Equal?(x=w310, y="False") -> (x != y?=w313:bool)
        n104 = Bundle By Name(cluster=w307, "NameDisplay"=w309) -> (w308:T5)
        n105 = case shown="True" w313 {
          tunnel: ["Face ID: Initialize Grab Image" "Face ID: Control Panel"] -> w320
          frame False {
            n106 = local write "Tab Control"(enum32{"Page 1", "Page 2", "Page 3"}."Page 1" ("Tab Control")) -> ()
            n107 = Two Button Dialog(message="Login Failed! Please try again to use the app.") -> ()  [unwired: 2 in, 1 out]
          }
          frame True {
            w329 = "Login Successful! Now you can use the app"  # Komunikat
            n108 = local write "Tab Control"(enum32{"Page 1", "Page 2", "Page 3", "Page 4"}."Page 3" ("Tab Control")) -> ()
            n109 = One Button Dialog(message=w329) -> ()  [unwired: 1 in, 1 out]
          }
        }
        n110 = call <vilib>:"Add State(s) to Queue__JKI_lib_State_Machine.vi"("State(s) in Front (\"\")"=w320, "State(s) in (\"\")"=w322) -> ("States Out"=w321:string)  [unwired: 13 in]
      }
      frame "Face ID: Control Panel" {
        n111 = control-ref of="Exit Application"() -> (w335:refnum<vi>)
        n112 = Unbundle By Name(w334) -> ("NameDisplay"=w331:string)
        n113 = event shown="[2] \"Manage input data\": Value Change" {
          selector: _ -> [_ _ _ _]
          dyn-events: _ -> [_ _ _ _]
          timeout: _ -> [_ _ _ _]
          tunnel: [_ "Macro: Exit" "Face ID: Control Panel" "Add User: Input Image Init"] -> w337
          tunnel: "Add user" -> [_ _ _ _]
          tunnel: w335 -> [_ _ _ _]
          tunnel: "Manage input data" -> [_ _ _ _]
          tunnel: w332 -> [_ _ w345 _]
          tunnel: w331 -> [_ _ w344 _]
          tunnel: [_ _ w343 _] -> w330
          event Timeout {
            n114 = event-data() -> ()  [unwired: 1 in, 3 out]
          }
          event "Exit Application": Value Change {
            n115 = event-data() -> ()  [unwired: 1 in, 6 out]
          }
          event "Manage input data": Value Change {
            # "Uaktualnienie danych w bazie danych"
            n116 = event-data() -> ()  [unwired: 1 in, 6 out]
            n117 = call "DatabaseUpdate.vi"("Input"="Input", "error in (no error)"=w345, "Imie"=w344) -> ("error out"=w343:errorcluster)  [unwired: 8 in]
          }
          event "Add user": Value Change {
            n118 = event-data() -> ()  [unwired: 1 in, 6 out]
            n119 = local write "Tab Control"(enum32{"Page 1", "Page 2", "Page 3", "Page 4"}."Page 4" ("Tab Control")) -> ()
          }
        }
        n120 = call <vilib>:"Add State(s) to Queue__JKI_lib_State_Machine.vi"("State(s) in Front (\"\")"=w337, "State(s) in (\"\")"=w338) -> ("States Out"=w339:string)  [unwired: 13 in]
      }
      frame "----------- Control -----------" {
      }
      frame "Control Panel: Add User" {
        n121 = Unbundle By Name(w354) -> ()  [unwired: 1 out]
      }
      frame "-------------- Add User ----------" {
      }
      frame "Add User: Input Image Init" {
        # "Korzystając z bloku \"Bundle by Name\" tworzony jest klaster złożony z referencji do obrazu oraz sesji kamery.\nDane te są przesyłane do kolejnych stanów za pomocą linii \"Data Wire\""
        # "Po zatwierdzeniu wyboru kamery blok sprawdza poprawność i dostępność kamery - na tej podstawie wykonuje się odpowiedni Case struktury"
        # "/// Blok opcjonalny\nWyświetla i pozwala wybrać jedną z dostępnych kamer"
        n122 = call "List Available Cameras.vi"("error in"=w366) -> ("error out"=w376:errorcluster, "VendorName"=w377:string[], "Available Cameras"=w378:string[])  [unwired: 8 in]
        n123 = call "Select Camera Dialog.vi"("error in (no error)"=w376, "Vendor Name"=w377, "Camera Name"=w378) -> ("error out"=w372:errorcluster, "No camera?"=w375:bool, "Interface Name"=w374:string)  [unwired: 6 in]
        n124 = case shown="False" w375 {
          tunnel: w374 -> [w389 _]
          tunnel: [w387 T4 refnum ("Session Out")] -> w373
          tunnel: w372 -> [w385 w394]
          tunnel: [w384 w394] -> w365
          tunnel: [w380 w392] -> w371
          tunnel: [w382 T1 refnum ("New Image")] -> w370
          tunnel: ["Add User: Grab Input Image" ("Remaining States") w392] -> w369
          tunnel: [10 w391] -> w363
          tunnel: w368 -> [_ w391]
          tunnel: w367 -> [w380 _]
          frame False {
            w390 = u32 5  # Number of Buffers
            n125 = call <vilib>:"IMAQdx Open Camera.vi"("error in"=w385, "Session In"=w389) -> ("error out"=w386:errorcluster, "Session Out"=w388:T4)  [unwired: 1 in, 7 out]
            n126 = call <vilib>:"IMAQdx Configure Grab.vi"("error in"=w386, "Number of Buffers"=w390, "Session In"=w388) -> ("error out"=w384:errorcluster, "Session Out"=w387:T4)  [unwired: 7 in]
            n127 = call "IMAQ Create"("Image Name"="Acquire Most Recent Image") -> ("New Image"=w382:T1)  [unwired: 3 in, 2 out]
          }
          frame True {
            w392 = ""
            # "Kasujemy kolejne stany.\n! I tak \"idzie\" do \"Error Handler\"."
            # "Generuje bBd: -1074360311"
            # "Camera not found"
          }
        }
        n128 = Bundle By Name(cluster=w362, "New Image"=w370, "IMAQdx Session"=w373) -> (w361:T5)
        n129 = call <vilib>:"Add State(s) to Queue__JKI_lib_State_Machine.vi"("State(s) in Front (\"\")"=w369, "State(s) in (\"\")"=w371) -> ("States Out"=w364:string)  [unwired: 13 in]
      }
      frame "Add User: Grab Input Image" {
        w403 = ".jpg"  # Rozszerzenie pliku
        # "Zapisanie danych nowego użytkownika \nw bazie danych"
        # "Konkatenacja trzech zmiennych typu string w celu \nutworzenia nazwy pliku"
        n130 = Unbundle By Name(w411) -> ("IMAQdx Session"=w417:T4, "New Image"=w416:T1)
        n131 = call "Take Image Case Struct.vi"("error in (no error)"=w409, "OK Button"="Save biometrics", "Image In"=w416, "Session In"=w417) -> ("error out"=w402:errorcluster, "State"=w408:string, "Image Out"=w414:T1, "Session Out"=w415:T4)  [unwired: 4 in]
        "Image Display 2" <- w414
        n132 = Concatenate Strings("Name", "Surname", w403) -> (w396:string)
        n133 = Equal?(x=w408, y="Face ID: Stop Grab Image") -> (x = y?=w406:bool)
        n134 = Bundle By Name(cluster=w411, "IMAQdx Session"=w415, "New Image"=w414, "Img Path"=w396) -> (w412:T5)
        n135 = Select(t="Add User: Stop Grab Image", s=w406, f="Event Structure\nAdd User: Grab Input Image") -> (s? t:f=w399:string)
        n136 = call <vilib>:"Add State(s) to Queue__JKI_lib_State_Machine.vi"("State(s) in Front (\"\")"=w399, "State(s) in (\"\")"=w410) -> ("States Out"=w413:string)  [unwired: 13 in]
        n137 = call "DatabaseWrite SubVI.vi"("Input name of the new user"="Name", "String"=w399, "Input second name of the new user"="Surname", "Image path to the users biometrics"=w396, "error in (no error)"=w402) -> ("error out"=w401:errorcluster)  [unwired: 10 in]
      }
      frame "Add User: Stop Grab Image" {
        n138 = Current VI's Path() -> (path=w432:path)
        n139 = Unbundle By Name(w429) -> ("Img Path"=w423:string, "New Image"=w433:T1, "IMAQdx Session"=w437:T4)
        n140 = Concatenate Strings("..\\Data\\Registered_Users\\", w423) -> (w421:string)
        n141 = String To Path(string=w421) -> (path=w420:path)
        n142 = call <vilib>:"IMAQdx Stop Acquisition.vi"("error in"=w419, "Session In"=w437) -> ("error out"=w441:errorcluster, "Session Out"=w440:T4)  [unwired: 8 out]
        n143 = call <vilib>:"IMAQdx Unconfigure Acquisition.vi"("error in"=w441, "Session In"=w440) -> ("error out"=w438:errorcluster, "Session Out"=w439:T4)  [unwired: 8 out]
        n144 = Build Path(base path=w432, name or relative path=w420) -> (appended path=w431:path)
        n145 = call <vilib>:"IMAQdx Close Camera.vi"("error in"=w438, "Session In"=w439) -> ("error out"=w435:errorcluster)  [unwired: 9 out]
        n146 = call-poly "IMAQ Write File 2"("error in (no error)"=w435, "File Path"=w431, "Image"=w433) -> ("error out"=w434:errorcluster)  [unwired: 7 in, 1 out]
        n147 = call "Imaq Dispose"("Image"=w433, "error in (no error)"=w434) -> ("error out"=w427:errorcluster)  [unwired: 4 in]
        n148 = Bundle By Name(cluster=w429, "IMAQdx Session"=T4 refnum) -> (w425:T5)
        n149 = call <vilib>:"Add State(s) to Queue__JKI_lib_State_Machine.vi"("State(s) in Front (\"\")"="Face ID: Control Panel", "State(s) in (\"\")"=w428) -> ("States Out"=w424:string)  [unwired: 13 in]
      }
    }
  }
